vi "4275A_Auto_Soak_On.vi"(8 "error in":errorcluster, 9 "Device Type":string) -> (0 "error out":errorcluster, 2 "Soak Time":dbl)   [LabVIEW 2020]
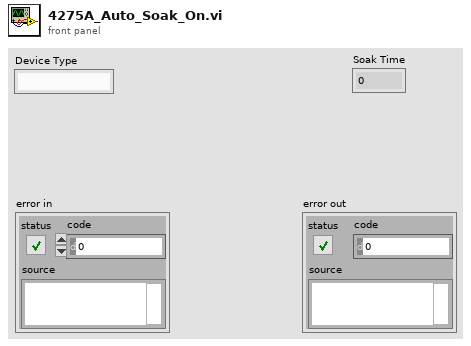
[diagram p1: front panel]
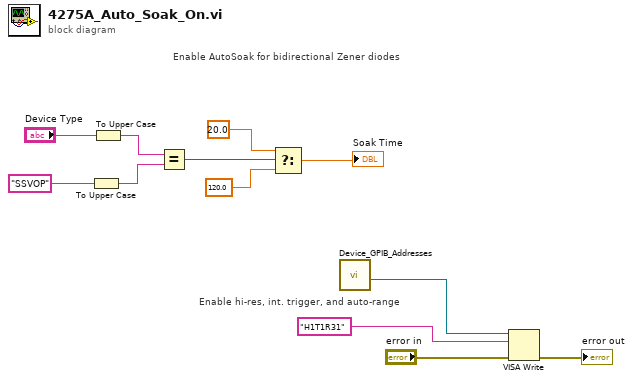
[diagram p0: block diagram]
diagram:
  # "Enable hi-res, int. trigger, and auto-range"
  # "Enable AutoSoak for bidirectional Zener diodes"
  n1 = To Upper Case(1:"SSVOP" ("string")) -> (0:w9:string)
  n2 = To Upper Case(1:"Device Type") -> (0:w10:string)
  n3 = Equal?(x=w10, y=w9) -> (x = y?=w8:bool)
  n4 = Select(t=20.0, s=w8, f=120.0) -> (s? t:f=→"Soak Time":dbl)
  n5 = call "Device_GPIB_Addresses.vi"() -> ("HP 4275A Address"=w4:refnum<visa-resource-name>)  [unwired: 9 in, 2 out]
  n6 = VISA Write(VISA resource name=w4, write buffer="H1T1R31" ("data"), error in (no error)="error in") -> (error out=→"error out":errorcluster)  [unwired: 2 out]
